vi "Get Time String.vi"(8 "error in (no error)":errorcluster, 11 "Offset (s)":i32) -> (0 "error out":errorcluster, 3 "Time String":string)   [LabVIEW 2024]
doc: "Gets the string of time."
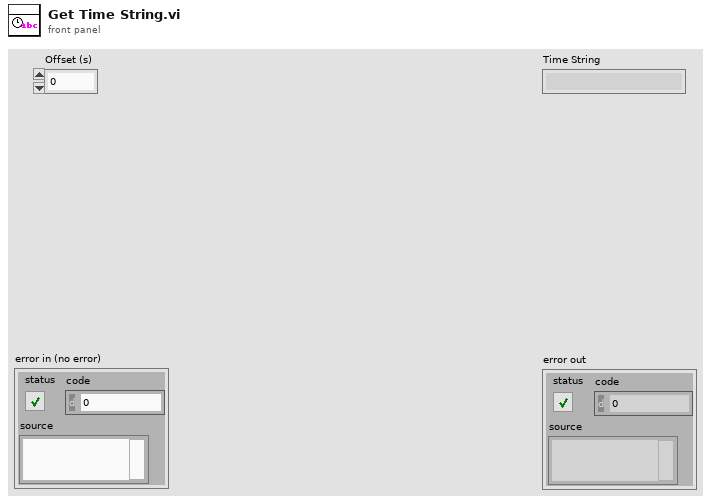
[diagram p1: front panel]
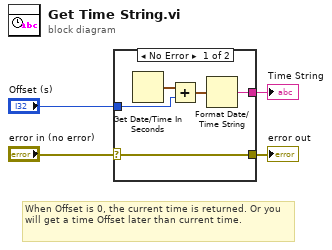
[diagram p0: block diagram]
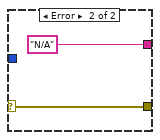
[diagram p2: hidden frame]
diagram:
  # "When Offset is 0, the current time is returned. Or you will get a time Offset later than current time."
  n1 = case shown="No Error" "error in (no error)" {
    selector: "error in (no error)" -> [w5 w11]
    tunnel: [w5 w11] -> w3
    tunnel: [w7 "N/A" ("date/time string")] -> w2
    tunnel: "Offset (s)" -> [w6 _]
    frame No Error {
      n2 = Get Date/Time In Seconds() -> (seconds since 1Jan1904=w9:timestamp)
      n3 = Add(x=w9, y=w6) -> (x+y=w8:timestamp)
      n4 = Format Date/Time String(seconds (now)=w8) -> (date/time string=w7:string)  [unwired: 2 in]
    }
    frame Error {
    }
  }
  "error out" <- w3
  "Time String" <- w2
